vi "store class data.vi"(7 "parent class":refnum<class>, 8 "error in":errorcluster, 10 "child class":refnum<class>, 11 "refnum in":T1) -> (0 "error out":errorcluster, 3 "refnum out":T1)   [LabVIEW 2020, in "Publisher Subscriber.lvlib"]
uses:
  Publisher Subscriber.lvlib
  Controls/node refnum.ctl
  Controls/node dvr data.ctl
  Controls/data cluster.ctl
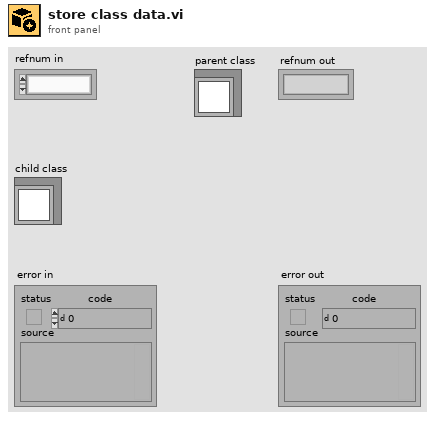
[diagram p1: front panel]
types:
  T1 = typedef "Publisher Subscriber.lvlib/node refnum.ctl" = refnum<k1>
  T2 = cluster{"Classes Map":map{string, refnum<class>}, "Name List[]":string[]}
  T3 = typedef "Publisher Subscriber.lvlib/node dvr data.ctl" = cluster{"queue ref":refnum<queue>, "subscription map ref":refnum<data-value>, "Command":string, "Data":variant, "Subscriptions []":set{string}, "variable dvr refs":refnum<data-value>}
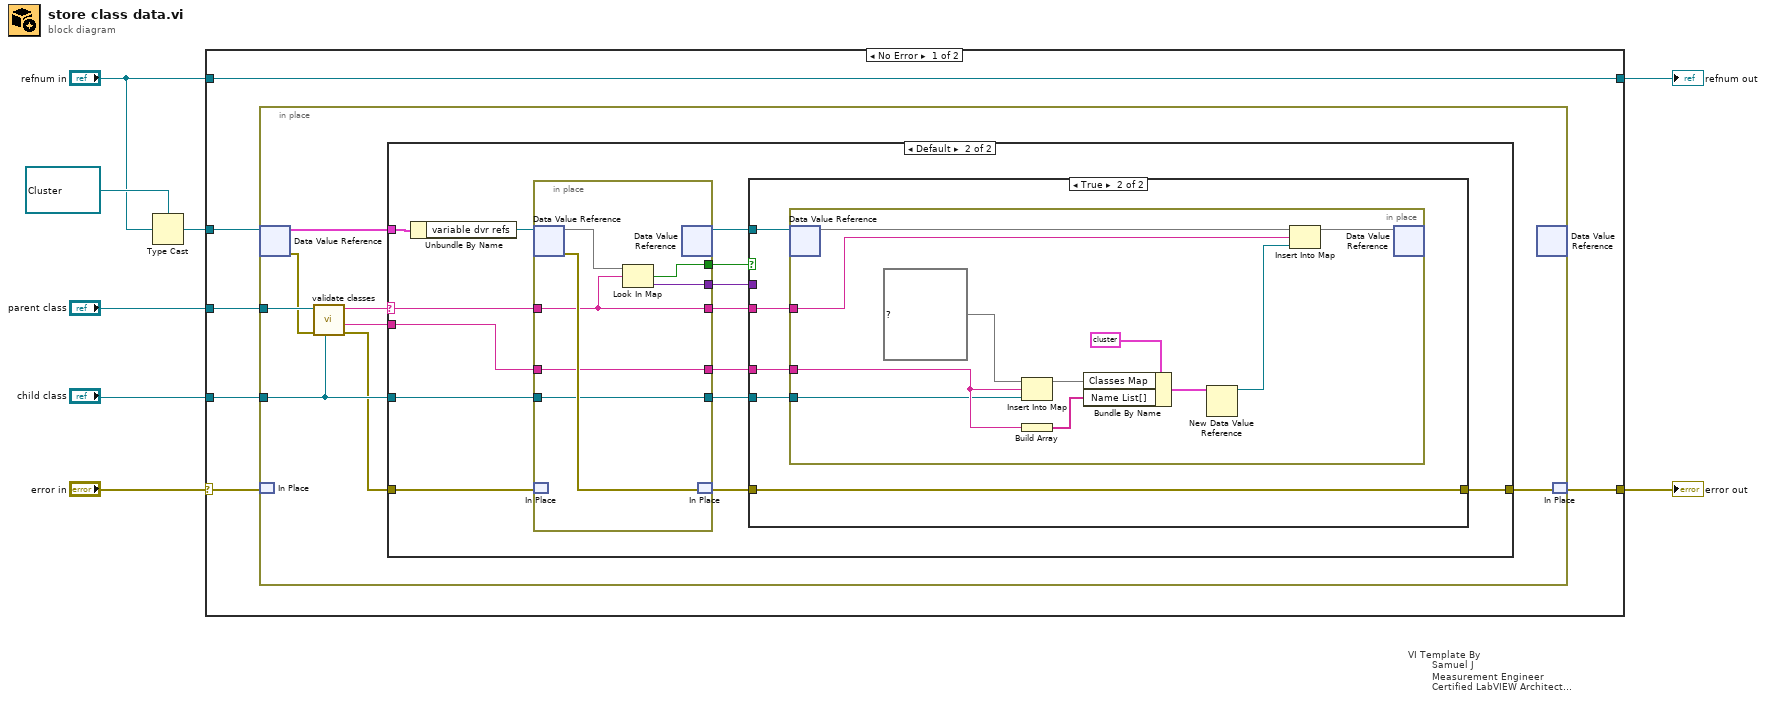
[diagram p0: block diagram]
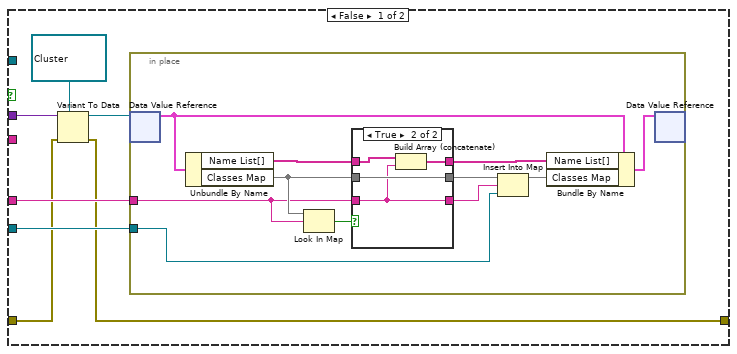
[diagram p3: hidden frame]
diagram:
  n1 = Type Cast(type=refnum<data-value> refnum ("data value reference"), x="refnum in") -> (*(type *) &x=w5:refnum<data-value>)
  n2 = case "VI Template By\n        Samuel J\n        Measurement Engineer\n        Certified LabVIEW Architect\n        Vestas Technology R&D Chennai" shown="No Error" "error in" {
    selector: "error in" -> [w12 w87]
    tunnel: [w11 w87] -> w7
    tunnel: w5 -> [w13 _]
    tunnel: [w14 w86] -> w4
    tunnel: "refnum in" -> [w14 w86]
    tunnel: "parent class" -> [w10 _]
    tunnel: "child class" -> [w9 _]
    frame No Error {
      n3 = in-place {
        in-place-border: w10 -> [w17]
        in-place-border: w9 -> [w20]
        n4 = in-place-dvr #1(w13) -> (w22:T3, w15:errorcluster)
        n5 = in-place-match #2(w12) -> ()  [unwired: 1 out]
        n6 = call "validate classes.vi"("Child"=w20, "error in"=w15, "Parent"=w17) -> ("error out"=w16:errorcluster, "class name"=w18:string, "unique parent name"=w19:string)  [unwired: 6 in]
        n7 = case shown="Default" w19 {
          selector: w19 -> [_ w32]
          tunnel: w22 -> [_ w37]
          tunnel: [w23 w25] -> w21
          tunnel: w20 -> [_ w35]
          tunnel: w16 -> [w23 w34]
          tunnel: w18 -> [_ w33]
          frame "" {
          }
          frame Default {
            n8 = Unbundle By Name(w37) -> ("variable dvr refs"=w36:refnum<data-value>)
            n9 = in-place {
              in-place-border: w32 -> [w81]
              in-place-border: w35 -> [w83]
              in-place-border: w33 -> [w82]
              in-place-border: [w83] -> w31
              in-place-border: [w82] -> w30
              in-place-border: [w81] -> w29
              in-place-border: [w80] -> w28
              in-place-border: [w79] -> w24
              n10 = in-place-dvr #3(w36) -> (w84:map{string, variant}, w85:errorcluster)
              n11 = in-place-match #4(w34) -> ()  [unwired: 1 out]
              n12 = Look In Map(map=w84, key=w81) -> (key not found?=w79:bool, value=w80:variant)  [unwired: 1 in]
              n13 = in-place-dvr #3() -> (w27:refnum<data-value>)  [unwired: 1 in, 1 out]
              n14 = in-place-match #4(w85) -> (w26:errorcluster)
            }
            n15 = case shown="True" w24 {
              tunnel: w31 -> [w44 w65]
              tunnel: w30 -> [w43 w66]
              tunnel: w29 -> [_ w64]
              tunnel: w28 -> [w42 _]
              tunnel: w27 -> [_ w67]
              tunnel: w26 -> [w40 w63]
              tunnel: [w39 w63] -> w25
              frame False {
                n16 = Variant To Data(error in=w40, type=refnum<data-value> refnum ("data value reference"), Variant=w42) -> (data=w41:refnum<data-value>, error out=w39:errorcluster)
                n17 = in-place {
                  in-place-border: w44 -> [w47]
                  in-place-border: w43 -> [w46]
                  n18 = in-place-dvr #5(w41) -> (w55:T2)  [unwired: 1 out]
                  n19 = Unbundle By Name(w55) -> ("Name List[]"=w52:string[], "Classes Map"=w51:map{string, refnum<class>})
                  n20 = Look In Map(map=w51, key=w46) -> (key not found?=w54:bool)  [unwired: 1 in, 1 out]
                  n21 = case shown="True" w54 {
                    tunnel: [w58 w60] -> w53
                    tunnel: w52 -> [w58 w61]
                    tunnel: w51 -> [w57 w62]
                    tunnel: [w57 w62] -> w49
                    tunnel: w46 -> [w56 w59]
                    tunnel: [w56 w59] -> w45
                    frame False {
                    }
                    frame True {
                      n22 = Build Array (concatenate)(w61, w59) -> (w60:string[])
                    }
                  }
                  n23 = Insert Into Map(map in=w49, key=w45, value=w47) -> (map out=w48:map{string, refnum<class>})  [unwired: 2 out]
                  n24 = Bundle By Name(cluster=w55, "Name List[]"=w53, "Classes Map"=w48) -> (w50:T2)
                  n25 = in-place-dvr #5(w50) -> ()  [unwired: 2 out]
                }
              }
              frame True {
                n26 = in-place {
                  in-place-border: w66 -> [w73]
                  in-place-border: w65 -> [w72]
                  in-place-border: w64 -> [w69]
                  n27 = in-place-dvr #6(w67) -> (w71:map{string, variant})  [unwired: 1 out]
                  n28 = Insert Into Map(map in=map{string, refnum<class>} {} ("Classes Map"), key=w73, value=w72) -> (map out=w76:map{string, refnum<class>})  [unwired: 2 out]
                  n29 = Build Array(w73) -> (w75:string[])
                  n30 = Bundle By Name(cluster=T2 {"Classes Map"={}, "Name List[]"=[]} ("Cluster"), "Classes Map"=w76, "Name List[]"=w75) -> (w74:T2)
                  n31 = New Data Value Reference(data value=w74) -> (data value reference=w68:refnum<data-value>)  [unwired: 1 in, 1 out]
                  n32 = Insert Into Map(map in=w71, key=w69, value=w68) -> (map out=w70:map{string, variant})  [unwired: 2 out]
                  n33 = in-place-dvr #6(w70) -> ()  [unwired: 2 out]
                }
              }
            }
          }
        }
        n34 = in-place-dvr #1() -> ()  [unwired: 1 in, 2 out]
        n35 = in-place-match #2(w21) -> (w11:errorcluster)
      }
    }
    frame Error {
    }
  }
  "error out" <- w7
  "refnum out" <- w4
